vi "Main.vi"() -> ()   [LabVIEW 2014, in "Configurable.lvlib"]
doc: "This template is based off of the Queued Message Handler design pattern and the Queued Message Handler project template that ships with LabVIEW.\n\nThe main difference is that the queue is private to this module and communication between modules is performed via Broadcast and Request events.\n\nRequest events are wrapped in public API methods and are handled in the Event Handling Loop (EHL) of this VI. Any module can register for Broadcast events sent by this module. The EHL generates messages based on user interface actions.\n\nThe Message Handling Loop (MHL) processes messages generated by the EHL, or by other messages. The messages are string values, so new messages can be added easily to the Message Cases case structure in the MHL. Each message cluster can also provide an optional value for Message Data, which is a variant that can be converted to whatever message-specific data is required.\n_____\nBased on Delacor QMH Project Template 4.0.0.47."
uses:
  Configurable.lvlib
  <vilib>/Delacor/Delacor QMH/Libraries/Cloneable Module Admin_class/Delacor_lib_QMH_Cloneable Module Admin.lvclass
  <vilib>/LabVIEW Open Source/Configuration Manager/Manager/ConfigManager.lvclass
  <vilib>/LabVIEW Open Source Project/Unicity/UniqueName/UniqueNameClass/UniqueName.lvclass
  ModuleConfiguration--Cluster.ctl
  Module Data--cluster.ctl
  <vilib>/Delacor/Delacor QMH/Libraries/Cloneable Module Admin_class/Delacor_lib_QMH_Cloneable Module Admin.lvclass/Delacor_lib_QMH_Cloneable Module Admin.ctl
  Stop Argument--cluster.ctl
  <vilib>/Delacor/Delacor QMH/Libraries/Module Admin_class/Delacor_lib_QMH_Module Admin.lvclass/Delacor_lib_QMH_Module Admin.ctl
  GetQualifiedName Argument--cluster.ctl
  GetQualifiedName (Reply Payload)--cluster.ctl
  GetConfiguration Argument--cluster.ctl
  GetConfiguration (Reply Payload)--cluster.ctl
  Modify Configuration Argument--cluster.ctl
  <vilib>/Utility/miscctls.llb/LVPointTypeDef.ctl
  <vilib>/LabVIEW Open Source Project/Unicity/UniqueName/UniqueNameClass/UniqueName.lvclass/UniqueName.ctl
  <vilib>/Delacor/Delacor QMH/Libraries/Cloneable Module Admin_class/Delacor_lib_QMH_Get Module ID.vi
  <vilib>/Delacor/Delacor QMH/Libraries/Module Admin_class/Delacor_lib_QMH_Get External Launch.vi
  <vilib>/Delacor/Delacor QMH/Libraries/Message Queue_class/Delacor_lib_QMH_Enqueue Message (Single).vi
  <vilib>/Utility/error.llb/Error Cluster From Error Code.vi
  <vilib>/ErrorRing/Error Ring.xnode
  <vilib>/Delacor/Delacor QMH/Libraries/Message Queue_class/Delacor_lib_QMH_Message Queue.lvclass
  Clone Registration/Clone Registration.lvlib
panel:
  out "Initial Configuration":T1
  out "Current Configuration":T1
  in  "Self":refnum<class "UniqueName.lvclass">
  in  "CfgManager":refnum<class "ConfigManager.lvclass">
  in  "Simulate MHL Error":bool
  in  "Simulate EHL Error":bool
  out "error out":errorcluster
  in  "Module Admin":refnum<class "Delacor_lib_QMH_Cloneable Module Admin.lvclass">
  out "Status":string
  # "Do not modify these nodes"
  # "This template is for the a Configurable  Delacor Queued Message Handler design pattern.\n\nSee the block diagram for more information on how to use this template.\nOther QMH Modules communicate with this Module via its Public API (wrappers for its Request Events).\n\nThis Module communicates with other Modules via its Broadcast Events.\nAny module that wants to get these messages, just registers for this module's Broadcast events."
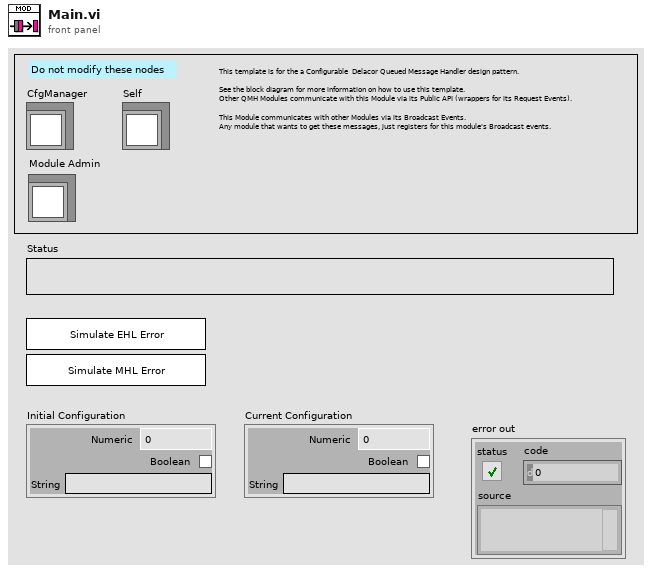
[diagram p1: front panel]
types:
  T1 = typedef "Configurable.lvlib/ModuleConfiguration--Cluster.ctl" = cluster{"Numeric":dbl, "Boolean":bool, "String":string}
  T2 = typedef "Configurable.lvlib/Module Data--cluster.ctl" = cluster{"Status":string, "CfgManager":refnum<class "ConfigManager.lvclass">, "Self":refnum<class "UniqueName.lvclass">}
  T3 = typedef "Configurable.lvlib/Request Events--cluster.ctl" = cluster{"Stop Module":refnum<user-event>, "Show Panel":refnum<user-event>, "Hide Panel":refnum<user-event>, "Show Diagram":refnum<user-event>, "Get Module Execution Status":refnum<user-event>, "GetQualifiedName":refnum<user-event>, "GetConfiguration":refnum<user-event>, "Modify Configuration":refnum<user-event>}
  T4 = enum32{"invalid lock state", "Not Locked", "Locked (No Password)", "Password-protected"}
  T5 = typedef "Configurable.lvlib/Stop Argument--cluster.ctl" = cluster{"Origin":string, "Module ID":i32, "Exit via Stop Module Req?":bool, "Wait for Module to stop?":bool}
  T6 = typedef "Configurable.lvlib/GetQualifiedName Argument--cluster.ctl" = cluster{"Module ID":i32, "Fully Qualified Name":string, "Wait Notifier":refnum<notifier>}
  T7 = typedef "Configurable.lvlib/GetConfiguration Argument--cluster.ctl" = cluster{"Module ID":i32, "Wait Notifier":refnum<notifier>}
  T8 = typedef "Configurable.lvlib/Modify Configuration Argument--cluster.ctl" = cluster{"Module ID":i32, "Configuration":T1}
  T9 = typedef "LVPointTypeDef.ctl" = cluster{"Horizontal":i16, "Vertical":i16}
  T10 = enum32{"Invalid", "Standard", "Closed", "Hidden", "Minimized", "Maximized"}
  T11 = typedef "Configurable.lvlib/GetQualifiedName (Reply Payload)--cluster.ctl" = cluster{"Fully Qualified Name":string, "GetQualifiedName_error":errorcluster}
  T12 = typedef "Configurable.lvlib/GetConfiguration (Reply Payload)--cluster.ctl" = cluster{"Configuration":T1, "GetConfiguration_error":errorcluster}
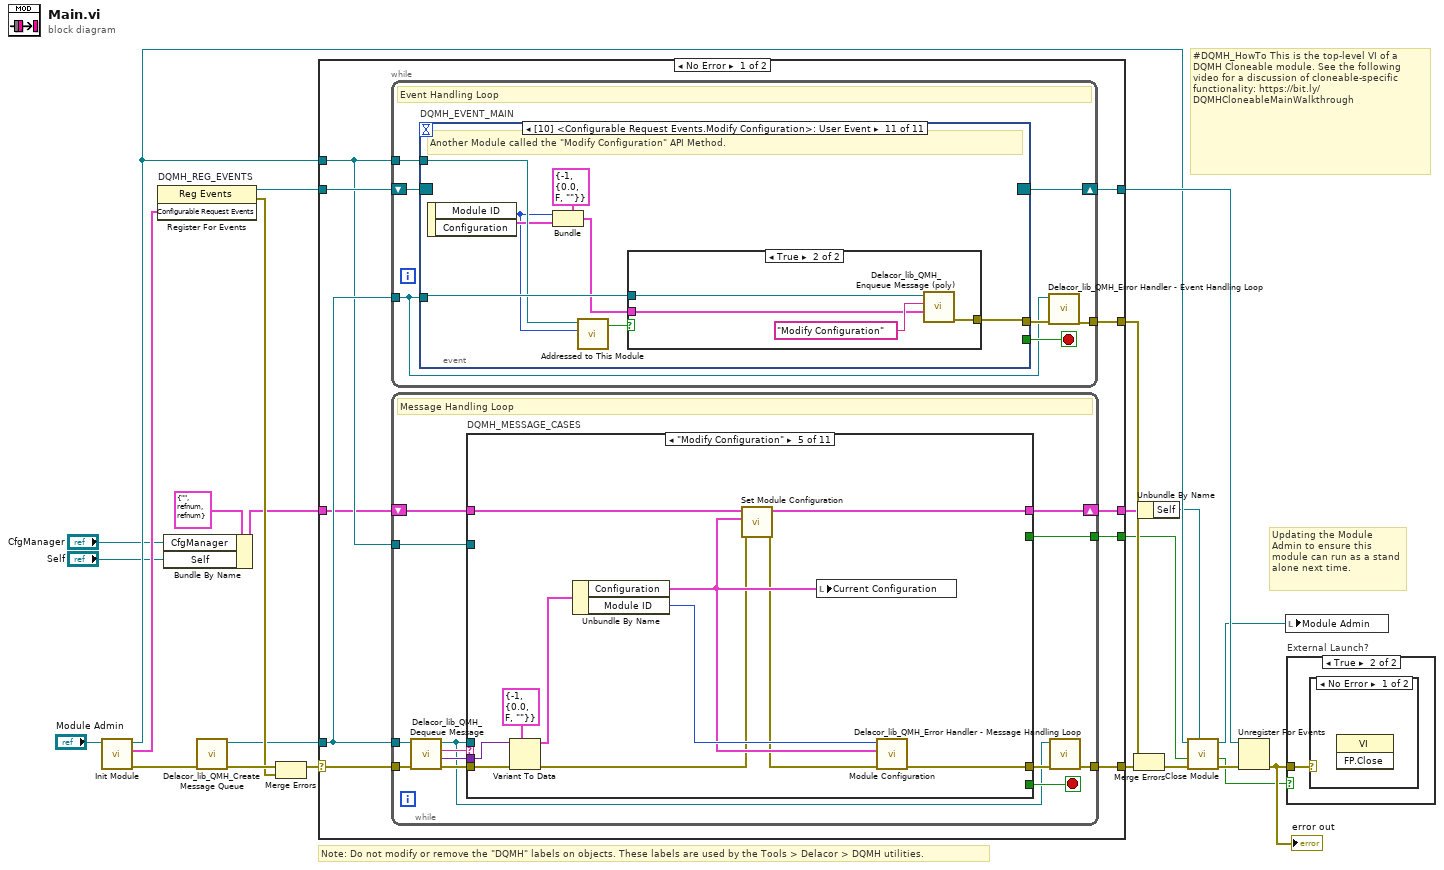
[diagram p0: block diagram]
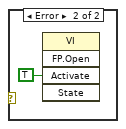
[diagram p3: hidden frame]
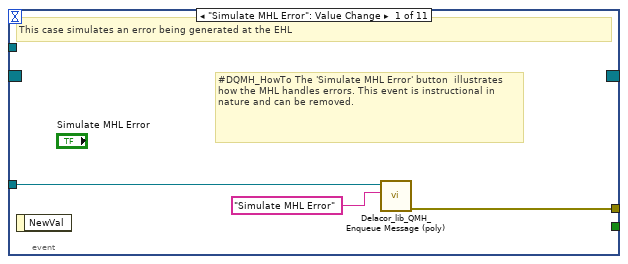
[diagram p4: hidden frame]
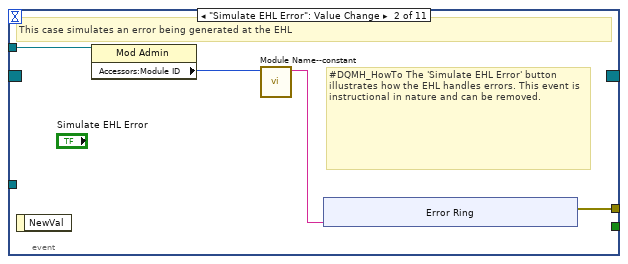
[diagram p5: hidden frame]
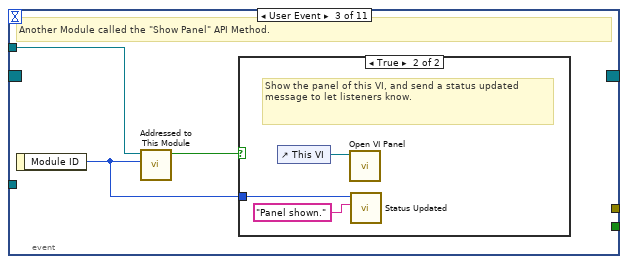
[diagram p6: hidden frame]
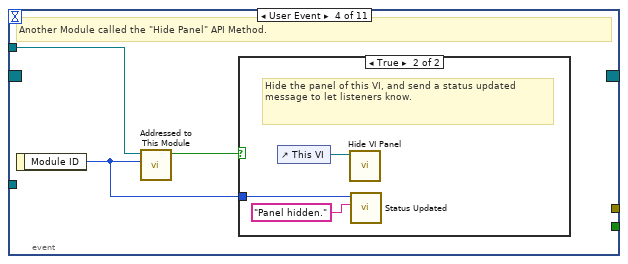
[diagram p8: hidden frame]
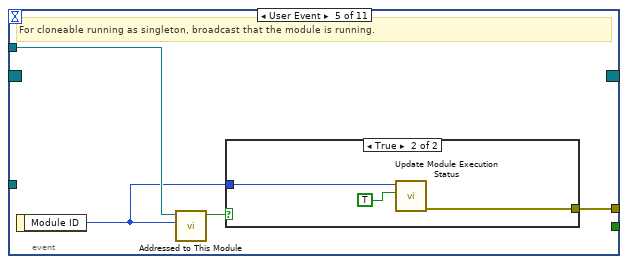
[diagram p10: hidden frame]
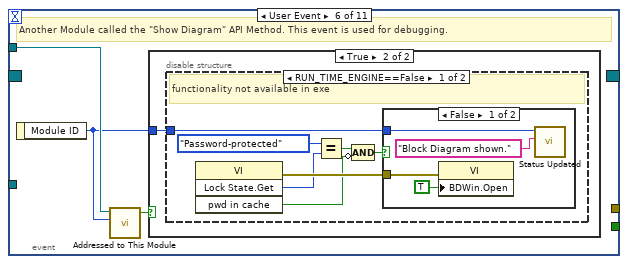
[diagram p12: hidden frame]
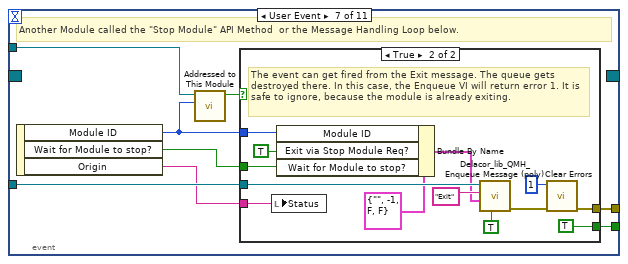
[diagram p16: hidden frame]
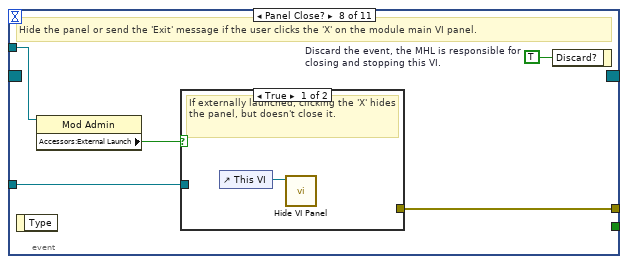
[diagram p18: hidden frame]
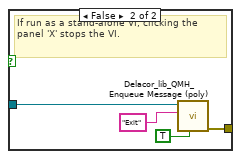
[diagram p19: hidden frame]
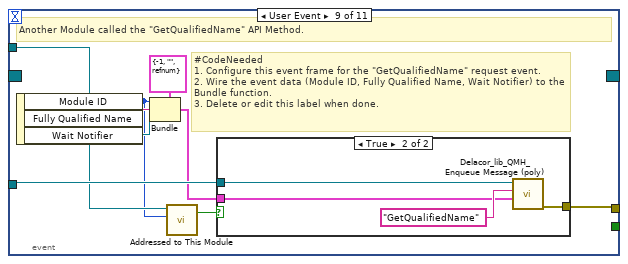
[diagram p20: hidden frame]
diagram:
  # "#DQMH_HowTo This is the top-level VI of a DQMH Cloneable module. See the following video for a discussion of cloneable-specific functionality: https://bit.ly/DQMHCloneableMainWalkthrough"
  # "Note: Do not modify or remove the \"DQMH\" labels on objects. These labels are used by the Tools > Delacor > DQMH utilities."
  # "Updating the Module Admin to ensure this module can run as a stand alone next time."
  n1 = call "Init Module.vi"("Cloneable Module Admin in"="Module Admin") -> ("error out"=w21:errorcluster, "Configurable Request Events"=w13:T3, "Cloneable Module Admin out"=w10:refnum<class "Delacor_lib_QMH_Cloneable Module Admin.lvclass">)  [unwired: 8 in]
  n2 = register-events "DQMH_REG_EVENTS"(w13) -> (reference out=w14:refnum<event-registration>, error out=w16:errorcluster)  [unwired: 2 in]
  n3 = Bundle By Name(cluster=T2 {"Status"="", "CfgManager"=refnum, "Self"=refnum} ("Data Cluster"), "CfgManager"="CfgManager", "Self"="Self") -> (w4:T2)
  n4 = call <vilib>:"Delacor_lib_QMH_Create Message Queue.vi"("error in (no error)"=w21) -> ("error out"=w18:errorcluster, "Message Queue out"=w12:refnum<class "Delacor_lib_QMH_Message Queue.lvclass">)  [unwired: 9 in]
  n5 = Merge Errors(w18, w16) -> (w17:errorcluster)
  n6 = case shown="No Error" w17 {
    selector: w17 -> [w32 w317]
    tunnel: [w34 w317] -> w22
    tunnel: [w31 w316] -> w15
    tunnel: w14 -> [w30 w316]
    tunnel: w12 -> [w29 _]
    tunnel: [w33 _] -> w23
    tunnel: w10 -> [w28 w312]
    tunnel: [w27 _] -> w8
    tunnel: w4 -> [w26 w309]
    tunnel: [w25 w309] -> w2
    frame No Error {
      n7 = while {
        tunnel: w29 -> [w35]
        shift-right: [w38] -> w31
        shift-left: w30 -> [w39]
        tunnel: [w40] -> w33
        tunnel: w28 -> [w36]
        stop <- w37 stop-if-true
        # "Event Handling Loop"
        n8 = event "DQMH_EVENT_MAIN" shown="[10] <Configurable Request Events.Modify Configuration>: User Event" {
          selector: w39 -> [_ _ _ _ _ _ _ _ _ _ _]
          dyn-events: [_ _ _ _ _ _ _ _ _ _ _] -> w38
          timeout: _ -> [_ _ _ _ _ _ _ _ _ _ _]
          tunnel: [_ _ _ _ _ _ w93 _ _ _ _] -> w37
          tunnel: w35 -> [w43 _ _ _ _ _ w96 w112 w129 w141 w153]
          tunnel: [w44 w48 _ _ w71 _ w97 w115 w124 w136 w148] -> w41
          tunnel: w36 -> [_ w47 w57 w63 w69 w76 w95 w113 w127 w139 w151]
          event "Simulate MHL Error": Value Change {
            # "#DQMH_HowTo The 'Simulate MHL Error' button  illustrates how the MHL handles errors. This event is instructional in nature and can be removed."
            # "This case simulates an error being generated at the EHL"
            n9 = event-data() -> ()  [unwired: 1 in, 1 out]
            n10 = call-poly <vilib>:"Delacor_lib_QMH_Enqueue Message (poly).vi"("Message"="Simulate MHL Error", "Message Queue in"=w43) -> ("error out"=w44:errorcluster)  [unwired: 8 in, 1 out]
          }
          event "Simulate EHL Error": Value Change {
            # "#DQMH_HowTo The 'Simulate EHL Error' button  illustrates how the EHL handles errors. This event is instructional in nature and can be removed."
            # "This case simulates an error being generated at the EHL"
            n11 = event-data() -> ()  [unwired: 1 in, 1 out]
            n12 = property class="Mod Admin"(reference=w47) -> ("Accessors:Module ID"=w46:i32)  [unwired: 1 in, 2 out]
            n13 = call "Module Name--constant.vi"("Module ID"=w46) -> ("Module Name"=w45:string)  [unwired: 10 in]
            n14 = xnode "Error Ring"("parameter 0"=w45) -> ("error out"=w48:errorcluster)
          }
          event User Event {
            # "Another Module called the \"Show Panel\" API Method."
            n15 = event-data() -> ("Module ID"=w56:i32)  [unwired: 1 in]
            n16 = call "Addressed to This Module.vi"("Module ID from Argument"=w56, "Module Admin"=w57) -> ("Addressed to this instance?"=w58:bool)  [unwired: 8 in, 1 out]
            n17 = case shown="True" w58 {
              tunnel: w56 -> [_ w59]
              frame False {
              }
              frame True {
                # "Show the panel of this VI, and send a status updated message to let listeners know."
                n18 = control-ref of="This VI"() -> (w61:refnum<vi>)
                n19 = call "Open VI Panel.vi"("VI"=w61) -> ()  [unwired: 10 in, 1 out]
                n20 = call "Status Updated.vi"("Status"="Panel shown." ("format string"), "Module ID"=w59) -> ()  [unwired: 9 in, 1 out]
              }
            }
          }
          event User Event {
            # "Another Module called the \"Hide Panel\" API Method."
            n21 = event-data() -> ("Module ID"=w62:i32)  [unwired: 1 in]
            n22 = call "Addressed to This Module.vi"("Module ID from Argument"=w62, "Module Admin"=w63) -> ("Addressed to this instance?"=w64:bool)  [unwired: 8 in, 1 out]
            n23 = case shown="True" w64 {
              tunnel: w62 -> [_ w65]
              frame False {
              }
              frame True {
                # "Hide the panel of this VI, and send a status updated message to let listeners know."
                n24 = control-ref of="This VI"() -> (w67:refnum<vi>)
                n25 = call "Hide VI Panel.vi"("VI"=w67) -> ()  [unwired: 10 in, 1 out]
                n26 = call "Status Updated.vi"("Status"="Panel hidden." ("format string"), "Module ID"=w65) -> ()  [unwired: 9 in, 1 out]
              }
            }
          }
          event User Event {
            # "For cloneable running as singleton, broadcast that the module is running."
            n27 = event-data() -> ("Module ID"=w68:i32)  [unwired: 1 in]
            n28 = call "Addressed to This Module.vi"("Module ID from Argument"=w68, "Module Admin"=w69) -> ("Addressed to this instance?"=w70:bool)  [unwired: 8 in, 1 out]
            n29 = case shown="True" w70 {
              tunnel: [_ w74] -> w71
              tunnel: w68 -> [_ w73]
              frame False {
              }
              frame True {
                n30 = call "Update Module Execution Status.vi"("Running?"=TRUE, "Module ID"=w73) -> ("error out"=w74:errorcluster)  [unwired: 9 in]
              }
            }
          }
          event User Event {
            # "Another Module called the \"Show Diagram\" API Method. This event is used for debugging."
            n31 = event-data() -> ("Module ID"=w75:i32)  [unwired: 1 in]
            n32 = call "Addressed to This Module.vi"("Module ID from Argument"=w75, "Module Admin"=w76) -> ("Addressed to this instance?"=w77:bool)  [unwired: 8 in, 1 out]
            n33 = case shown="True" w77 {
              tunnel: w75 -> [_ w78]
              frame False {
              }
              frame True {
                n34 = disable-structure shown="RUN_TIME_ENGINE==False" {
                  disable-tunnel: w78 -> [w79 _]
                  frame condition #0 (active) {
                    # "functionality not available in exe"
                    n35 = invoke class="VI" method="Lock State.Get"() -> (error out=w85:errorcluster, "Get Lock State"=w84:T4, "pwd in cache"=w81:bool)  [unwired: 4 in, 1 out]
                    n36 = Equal?(x=T4."Password-protected", y=w84) -> (x = y?=w82:bool)
                    n37 = Compound Arithmetic op=AND(w82, invert w81) -> (w80:bool)
                    n38 = case shown="False" w80 {
                      tunnel: w85 -> [w89 _]
                      tunnel: w79 -> [w86 _]
                      frame False {
                        n39 = property class="VI"(error in=w89, "BDWin.Open"=TRUE ("Block Diagram Window:Open")) -> ()  [unwired: 1 in, 2 out]
                        n40 = call "Status Updated.vi"("Status"="Block Diagram shown." ("format string"), "Module ID"=w86) -> ()  [unwired: 9 in, 1 out]
                      }
                      frame True {
                        # "Password-protected VI, and the password is not in the cache. Do not show the diagram."
                      }
                    }
                  }
                  frame condition #1 {
                  }
                }
              }
            }
          }
          event User Event {
            # "Another Module called the \"Stop Module\" API Method  or the Message Handling Loop below."
            n41 = event-data() -> ("Module ID"=w91:i32, "Wait for Module to stop?"=w92:bool, "Origin"=w90:string)  [unwired: 1 in]
            n42 = call "Addressed to This Module.vi"("Module ID from Argument"=w91, "Module Admin"=w95) -> ("Addressed to this instance?"=w94:bool)  [unwired: 8 in, 1 out]
            n43 = case shown="True" w94 {
              tunnel: [_ w109] -> w97
              tunnel: w96 -> [_ w105]
              tunnel: [_ TRUE] -> w93
              tunnel: w92 -> [_ w100]
              tunnel: w91 -> [_ w102]
              tunnel: w90 -> [_ w98]
              frame False {
              }
              frame True {
                # "The event can get fired from the Exit message. The queue gets destroyed there. In this case, the Enqueue VI will return error 1. It is safe to ignore, because the module is already exiting."
                n44 = local write "Status"(w98) -> ()
                n45 = Bundle By Name(cluster=T5 {"Origin"="", "Module ID"=-1, "Exit via Stop Module Req?"=FALSE, "Wait for Module to stop?"=FALSE} ("Stop Argument"), "Module ID"=w102, "Exit via Stop Module Req?"=TRUE, "Wait for Module to stop?"=w100) -> (w99:T5)
                n46 = call-poly <vilib>:"Delacor_lib_QMH_Enqueue Message (poly).vi"("Priority Message? (F)"=TRUE, "Message Data"=w99, "Message"="Exit", "Message Queue in"=w105) -> ("error out"=w110:errorcluster)  [unwired: 6 in, 1 out]
                n47 = call <vilib>:"Clear Errors.vi"("error in (no error)"=w110, "specific error code to clear (0: all)"=1) -> ("error out"=w109:errorcluster)  [unwired: 4 in, 1 out]
              }
            }
          }
          event Panel Close? {
            w114 = TRUE  # Discard the event, the MHL is responsible for closing and stopping this VI.
            # "Hide the panel or send the 'Exit' message if the user clicks the 'X' on the module main VI panel."
            n48 = event-data() -> ()  [unwired: 1 in, 1 out]
            n49 = property class="Mod Admin"(reference=w113) -> ("Accessors:External Launch"=w111:bool)  [unwired: 1 in, 2 out]
            n50 = case shown="True" w111 {
              tunnel: w112 -> [_ w119]
              tunnel: [_ w120] -> w115
              frame True {
                # "If externally launched, clicking the 'X' hides the panel, but doesn't close it."
                n51 = control-ref of="This VI"() -> (w116:refnum<vi>)
                n52 = call "Hide VI Panel.vi"("VI"=w116) -> ()  [unwired: 10 in, 1 out]
              }
              frame False {
                # "If run as a stand-alone VI, clicking the panel 'X' stops the VI."
                n53 = call-poly <vilib>:"Delacor_lib_QMH_Enqueue Message (poly).vi"("Priority Message? (F)"=TRUE, "Message"="Exit", "Message Queue in"=w119) -> ("error out"=w120:errorcluster)  [unwired: 7 in, 1 out]
              }
            }
            n54 = event-data("Discard?"=w114) -> ()  [unwired: 1 in, 1 out]
          }
          event User Event {
            # "#CodeNeeded\n1. Configure this event frame for the \"GetQualifiedName\" request event.\n2. Wire the event data (Module ID, Fully Qualified Name, Wait Notifier) to the Bundle function.\n3. Delete or edit this label when done."
            # "Another Module called the \"GetQualifiedName\" API Method."
            n55 = event-data() -> ("Module ID"=w121:i32, "Fully Qualified Name"=w123:string, "Wait Notifier"=w122:refnum<notifier>)  [unwired: 1 in]
            n56 = Bundle(cluster=T6 {"Module ID"=-1, "Fully Qualified Name"="", "Wait Notifier"=refnum} ("GetQualifiedName Argument"), "Module ID"=w121, "Fully Qualified Name"=w123, "Wait Notifier"=w122) -> (w125:T6)
            n57 = call "Addressed to This Module.vi"("Module ID from Argument"=w121, "Module Admin"=w127) -> ("Addressed to this instance?"=w128:bool)  [unwired: 8 in, 1 out]
            n58 = case shown="True" w128 {
              tunnel: w129 -> [_ w133]
              tunnel: w125 -> [_ w131]
              tunnel: [_ w130] -> w124
              frame False {
              }
              frame True {
                n59 = call-poly <vilib>:"Delacor_lib_QMH_Enqueue Message (poly).vi"("Message Data"=w131, "Message"="GetQualifiedName", "Message Queue in"=w133) -> ("error out"=w130:errorcluster)  [unwired: 7 in, 1 out]
              }
            }
          }
          event User Event {
            # "Another Module called the \"GetConfiguration\" API Method."
            n60 = event-data() -> ("Module ID"=w134:i32, "Wait Notifier"=w135:refnum<notifier>)  [unwired: 1 in]
            n61 = Bundle(cluster=T7 {"Module ID"=-1, "Wait Notifier"=refnum} ("GetConfiguration Argument"), "Module ID"=w134, "Wait Notifier"=w135) -> (w137:T7)
            n62 = call "Addressed to This Module.vi"("Module ID from Argument"=w134, "Module Admin"=w139) -> ("Addressed to this instance?"=w140:bool)  [unwired: 8 in, 1 out]
            n63 = case shown="True" w140 {
              tunnel: w141 -> [_ w145]
              tunnel: w137 -> [_ w143]
              tunnel: [_ w142] -> w136
              frame False {
              }
              frame True {
                n64 = call-poly <vilib>:"Delacor_lib_QMH_Enqueue Message (poly).vi"("Message Data"=w143, "Message"="GetConfiguration", "Message Queue in"=w145) -> ("error out"=w142:errorcluster)  [unwired: 7 in, 1 out]
              }
            }
          }
          event User Event {
            # "Another Module called the \"Modify Configuration\" API Method."
            n65 = event-data() -> ("Module ID"=w146:i32, "Configuration"=w147:T1)  [unwired: 1 in]
            n66 = Bundle(cluster=T8 {"Module ID"=-1, "Configuration"={"Numeric"=0.0, "Boolean"=FALSE, "String"=""}} ("Modify Configuration Argument"), "Module ID"=w146, "Configuration"=w147) -> (w149:T8)
            n67 = call "Addressed to This Module.vi"("Module ID from Argument"=w146, "Module Admin"=w151) -> ("Addressed to this instance?"=w152:bool)  [unwired: 8 in, 1 out]
            n68 = case shown="True" w152 {
              tunnel: w153 -> [_ w157]
              tunnel: w149 -> [_ w155]
              tunnel: [_ w154] -> w148
              frame False {
              }
              frame True {
                n69 = call-poly <vilib>:"Delacor_lib_QMH_Enqueue Message (poly).vi"("Message Data"=w155, "Message"="Modify Configuration", "Message Queue in"=w157) -> ("error out"=w154:errorcluster)  [unwired: 7 in, 1 out]
              }
            }
          }
        }
        n70 = call-dynamic "Delacor_lib_QMH_Error Handler - Event Handling Loop.vi"("error in (no error)"=w41, "Message Queue in"=w35) -> ("dup error in"=w40:errorcluster)  [unwired: 8 in, 1 out]
      }
      n71 = while {
        tunnel: w29 -> [w161]
        shift-right: [w165] -> w25
        shift-left: w26 -> [w166]
        tunnel: w32 -> [w169]
        tunnel: [w167] -> w34
        tunnel: w28 -> [w159]
        tunnel: [w158] -> w27
        stop <- w164 stop-if-true
        # "Message Handling Loop"
        n72 = call-dynamic "Delacor_lib_QMH_Dequeue Message.vi"("error in (no error)"=w169, "Message Queue in"=w161) -> ("error out"=w168:errorcluster, "Message Data"=w162:variant, "Message"=w163:string, "Message Queue out"=w160:refnum<class "Delacor_lib_QMH_Message Queue.lvclass">)  [unwired: 6 in]
        n73 = case "DQMH_MESSAGE_CASES" shown="\"Modify Configuration\"" w163 {
          selector: w163 -> [_ _ _ _ _ _ _ _ _ _ w296]
          tunnel: w160 -> [_ _ _ _ _ _ _ w246 _ w286 _]
          tunnel: w168 -> [w197 w201 w217 w229 w240 w243 w245 w256 w269 w292 w298]
          tunnel: [w179 w201 w206 w221 w234 w242 w245 w252 w268 w289 w299] -> w170
          tunnel: w166 -> [w173 w200 w211 w220 w236 w241 w244 w251 w266 w285 w297]
          tunnel: [w189 w200 w211 w219 w235 w241 w244 w251 w266 w285 w297] -> w165
          tunnel: [_ _ _ _ _ _ _ _ _ w284 _] -> w164
          tunnel: w162 -> [_ _ w216 w228 w239 _ _ w250 _ w282 _]
          tunnel: w159 -> [w185 _ _ _ _ _ _ w249 w264 w278 w294]
          tunnel: [_ _ _ _ _ _ _ _ _ w280 _] -> w158
          frame "Initialize" {
            w183 = "Initial Message" ("Initial Message")
            # "THIS OVERRIDES THE\nCONFIG FOR DEMO PURPOSES.\nREMOVE IT."
            # "Initialize - Any operation that needs to be done before the module can receive messages. Synchronize Caller Events.vi will inform Start Module.vi that the module has launched and is ready to receive messages. Module Did Init.vi will broadcast that the module initialized."
            n74 = call "Synchronize Caller Events.vi"("error in (no error)"=w197, "Module Admin"=w185) -> ("error out"=w196:errorcluster, "Module Admin out"=w174:refnum<class "Delacor_lib_QMH_Cloneable Module Admin.lvclass">)  [unwired: 8 in]
            n75 = Unbundle By Name(w173) -> ("Self"=w172:refnum<class "UniqueName.lvclass">)
            n76 = call <vilib>:"Read UUID.vi"("UniqueName in"=w172) -> ("UUID"=w171:string)  [unwired: 9 in, 1 out]
            n77 = property class="Mod Admin"(reference=w174) -> ("Accessors:Module ID"=w178:i32, "Accessors:External Launch"=w186:bool)  [unwired: 1 in, 2 out]
            n78 = Random Number (0-1)() -> (number: 0 to 1=w182:dbl)
            n79 = call "Get Module Configuration.vi"("Data Cluster"=w173) -> ("Configuration"=w181:T1, "Data Cluster dup"=w177:T2)  [unwired: 8 in, 1 out]
            n80 = Bundle By Name(cluster=w181, "Numeric"=w182, "String"=w171) -> (w175:T1)
            "Initial Configuration" <- w175
            n81 = call "Module Name--constant.vi"("Module ID"=w178) -> ("Module Name"=w193:string)  [unwired: 10 in]
            n82 = local write "Current Configuration"(w175) -> ()
            n83 = call "Set Module Configuration.vi"("Configuration"=w175, "Data Cluster"=w177) -> ("Data Cluster dup"=w176:T2)  [unwired: 8 in, 1 out]
            n84 = call "Module Name--constant.vi"("Module ID"=w178) -> ("Module Name"=w187:string)  [unwired: 10 in]
            n85 = property class="VI"("Front Panel.Title"=w193) -> (reference out=w195:refnum<vi>, error out=w199:errorcluster)  [unwired: 2 in]
            n86 = Select(t=T10."Hidden" ("State"), s=w186, f=T10."Standard" ("State")) -> (s? t:f=w190:T10)
            n87 = call "Module Did Init.vi"("error in (no error)"=w196, "Initialized?"=TRUE, "Origin"=w187, "Module ID"=w178) -> ("error out"=w180:errorcluster)  [unwired: 7 in]
            n88 = invoke class="VI" method="FP.Open"(reference=w195, error in=w199, "State"=w190) -> (reference out=w194:refnum<vi>, error out=w198:errorcluster)  [unwired: 2 in, 3 out]
            n89 = Bundle By Name(cluster=w176, "Status"=w183) -> (w189:T2)
            n90 = invoke class="VI" method="FP.Center"(reference=w194, error in=w198) -> ()  [unwired: 1 in, 3 out]
            n91 = property on="Pane" class="Pane"("Origin"=T9 {"Horizontal"=0, "Vertical"=0}) -> ()  [unwired: 2 in, 2 out]
            n92 = call "Module Configuration.vi"("error in (no error)"=w180, "Configuration"=w175, "Module ID"=w178) -> ("error out"=w179:errorcluster)  [unwired: 8 in]
            "Status" <- w183
          }
          frame "--- Module Specific ---" {
            # "Separator -- The following cases handle messages specific to this Module."
          }
          frame "GetQualifiedName" {
            # "Requests the module's Fully Qualified Name"
            n93 = Unbundle By Name(w211) -> ("Self"=w210:refnum<class "UniqueName.lvclass">)
            n94 = Variant To Data(error in=w217, type=T6 {"Module ID"=-1, "Fully Qualified Name"="", "Wait Notifier"=refnum} ("GetQualifiedName Argument"), Variant=w216) -> (data=w214:T6, error out=w205:errorcluster)
            n95 = call <vilib>:"Read Fully Qualified Name.vi"("UniqueName in"=w210) -> ("Fully Qualified Name"=w204:string)  [unwired: 9 in, 1 out]
            n96 = Unbundle By Name(w214) -> ("Wait Notifier"=w212:refnum<notifier>, "Module ID"=w208:i32)
            n97 = Bundle By Name(cluster=T11 {"Fully Qualified Name"="", "GetQualifiedName_error"={"status"=FALSE, "code"=0, "source"=""}} ("GetQualifiedName (Reply Payload)"), "Fully Qualified Name"=w204) -> (w213:T11)
            n98 = Format Into String(format string="FQN: %s", w204) -> (resulting string=w203:string)  [unwired: 2 in, 1 out]
            n99 = Send Notification(notification=w213, notifier=w212, error in (no error)=w205) -> (error out=w207:errorcluster)  [unwired: 1 out]
            n100 = call "Status Updated.vi"("error in (no error)"=w207, "Status"=w203, "Module ID"=w208) -> ("error out"=w206:errorcluster)  [unwired: 8 in]
          }
          frame "GetConfiguration" {
            n101 = Variant To Data(error in=w229, type=T7 {"Module ID"=-1, "Wait Notifier"=refnum} ("GetConfiguration Argument"), Variant=w228) -> (data=w226:T7, error out=w222:errorcluster)
            n102 = call "Get Module Configuration.vi"("error in (no error)"=w222, "Data Cluster"=w220) -> ("error out"=w221:errorcluster, "Configuration"=w218:T1, "Data Cluster dup"=w219:T2)  [unwired: 7 in]
            "Current Configuration" <- w218
            n103 = Unbundle By Name(w226) -> ("Wait Notifier"=w225:refnum<notifier>)
            n104 = Bundle By Name(cluster=T12 {"Configuration"={"Numeric"=0.0, "Boolean"=FALSE, "String"=""}, "GetConfiguration_error"={"status"=FALSE, "code"=0, "source"=""}} ("GetConfiguration (Reply Payload)"), "Configuration"=w218, "GetConfiguration_error"=w221) -> (w224:T12)
            n105 = Send Notification(notification=w224, notifier=w225) -> ()  [unwired: 1 in, 2 out]
          }
          frame "Modify Configuration" {
            n106 = Variant To Data(error in=w240, type=T8 {"Module ID"=-1, "Configuration"={"Numeric"=0.0, "Boolean"=FALSE, "String"=""}} ("Modify Configuration Argument"), Variant=w239) -> (data=w237:T8, error out=w231:errorcluster)
            n107 = Unbundle By Name(w237) -> ("Configuration"=w232:T1, "Module ID"=w233:i32)
            n108 = call "Set Module Configuration.vi"("error in (no error)"=w231, "Configuration"=w232, "Data Cluster"=w236) -> ("error out"=w230:errorcluster, "Data Cluster dup"=w235:T2)  [unwired: 7 in]
            n109 = local write "Current Configuration"(w232) -> ()
            n110 = call "Module Configuration.vi"("error in (no error)"=w230, "Configuration"=w232, "Module ID"=w233) -> ("error out"=w234:errorcluster)  [unwired: 8 in]
          }
          frame "---Copy This Frame---" {
            # "Duplicate this frame when creating new messages.  Change this comment in the duplicated frame to describe this message."
            n111 = Merge Errors(w243) -> (w242:errorcluster)
          }
          frame "--- Exit and Error Handling---" {
            # "Separator - the following cases handle errors and exit messages."
          }
          frame "Error" {
            # "#CodeRecommended - If you ever change the name of this \"Error\" message, you'll need to update the name in the Check Loop Error.vi as well."
            # "#CodeRecommended - If the module is running in standalone mode (External Launch = FALSE), this code will pop up an error dialog and call the 'Exit' message if an error occurs. Add more fine-grained error handling here."
            # "Error - Check the error message data and respond accordingly. This message is sent by the \"Error Handler\" VIs at the end of each loop in this application."
            n112 = property class="Mod Admin"(reference=w249) -> ("Accessors:External Launch"=w247:bool, "Accessors:Module ID"=w248:i32)  [unwired: 1 in, 2 out]
            n113 = Variant To Data(error in=w256, type=errorcluster {"status"=FALSE, "code"=0, "source"=""} ("error constant"), Variant=w250) -> (data=w257:errorcluster, error out=w254:errorcluster)
            n114 = call "Error Reported.vi"("Error"=w257, "Module ID"=w248) -> ()  [unwired: 9 in, 1 out]
            n115 = case shown="False" w247 {
              tunnel: [w262 _] -> w253
              tunnel: w246 -> [w260 _]
              tunnel: w257 -> [w261 _]
              frame False {
                # "If the module is running standalone, then pop up an error dialog and call the \"Exit\" message."
                n116 = call <vilib>:"Simple Error Handler.vi"("error in (no error)"=w261) -> ()  [unwired: 4 in, 5 out]
                n117 = call-poly <vilib>:"Delacor_lib_QMH_Enqueue Message (poly).vi"("Priority Message? (F)"=TRUE, "Message"="Exit", "Message Queue in"=w260) -> ("error out"=w262:errorcluster)  [unwired: 7 in, 1 out]
              }
              frame True {
                # "If the module was launched externally, calling the Error Reported broadcast VI is the only action performed by the \"Error\" message. The module's caller can then process the error appropriately."
              }
            }
            n118 = Merge Errors(w254, w253) -> (w252:errorcluster)
            n119 = local write "error out"(w252) -> ()
          }
          frame "Simulate MHL Error" {
            # "#DQMH_HowTo The 'Simulate MHL Error' button  illustrates how the MHL handles errors. This event is instructional in nature and can be removed."
            # "Simulate an error occurring at the MHL"
            n120 = property class="Mod Admin"(reference=w264) -> ("Accessors:Module ID"=w265:i32)  [unwired: 1 in, 2 out]
            n121 = call "Module Name--constant.vi"("Module ID"=w265) -> ("Module Name"=w263:string)  [unwired: 10 in]
            n122 = xnode "Error Ring"("parameter 0"=w263) -> ("error out"=w267:errorcluster)
            n123 = Merge Errors(w269, w267) -> (w268:errorcluster)
          }
          frame "Exit" {
            w283 = 91  # 91: not all Exit messages will have an argument
            w284 = TRUE  # Stop the VI
            # "Release the message queue reference"
            # "#CodeNeeded - Add any required cleanup code here."
            # "Exit - Exit the application."
            n124 = Variant To Data(error in=w292, type=T5 {"Origin"="", "Module ID"=-1, "Exit via Stop Module Req?"=FALSE, "Wait for Module to stop?"=FALSE} ("Stop Argument"), Variant=w282) -> (data=w279:T5, error out=w287:errorcluster)
            n125 = call <vilib>:"Clear Errors.vi"("error in (no error)"=w287, "specific error code to clear (0: all)"=w283) -> ("error out"=w291:errorcluster)  [unwired: 4 in, 1 out]
            n126 = control-ref of="This VI"() -> (w277:refnum<vi>)
            n127 = call-dynamic "Delacor_lib_QMH_Release Message Queue.vi"("error in (no error)"=w291, "Message Queue"=w286) -> ("error out"=w290:errorcluster)  [unwired: 9 in]
            n128 = call "Handle Exit.vi"("Stop Argument"=w279, "Module Admin in"=w278, "VI reference"=w277) -> ("error out"=w288:errorcluster, "Wait for Stop?"=w280:bool)  [unwired: 7 in]
            n129 = Merge Errors(w290, w288) -> (w289:errorcluster)
          }
          frame Default {
            # "'Default' case only runs if there is a message that isn't defined in any of the other cases.  Output a programming error."
            n130 = property class="Mod Admin"(reference=w294) -> ("Accessors:Module ID"=w293:i32)  [unwired: 1 in, 2 out]
            n131 = call "Module Name--constant.vi"("Module ID"=w293) -> ("Module Name"=w295:string)  [unwired: 10 in]
            n132 = xnode "Error Ring"("parameter 0"=w296, "parameter 1"=w295) -> ("error out"=w300:errorcluster)
            n133 = Merge Errors(w298, w300) -> (w299:errorcluster)
          }
        }
        n134 = call-dynamic "Delacor_lib_QMH_Error Handler - Message Handling Loop.vi"("error in (no error)"=w170, "Message Queue in"=w160) -> ("dup error in"=w167:errorcluster)  [unwired: 8 in, 1 out]
      }
    }
    frame Error {
      n135 = call "Synchronize Caller Events.vi"("Module Admin"=w312) -> ("Module Admin out"=w311:refnum<class "Delacor_lib_QMH_Cloneable Module Admin.lvclass">)  [unwired: 9 in, 1 out]
      n136 = property class="Mod Admin"(reference=w311) -> ("Accessors:Module ID"=w310:i32)  [unwired: 1 in, 2 out]
      n137 = call "Module Name--constant.vi"("Module ID"=w310) -> ("Module Name"=w315:string)  [unwired: 10 in]
      n138 = call "Remove.vi"("Module ID"=w310) -> ()  [unwired: 9 in, 2 out]
      n139 = Format Into String(format string="An error occurred during initialization. %s is no longer running.", w315) -> (resulting string=w313:string)  [unwired: 2 in, 1 out]
      n140 = call "Error Reported.vi"("Additional Information"=w313, "Error"=w317, "Module ID"=w310) -> ()  [unwired: 8 in, 1 out]
    }
  }
  n141 = Merge Errors(w23, w22) -> (w24:errorcluster)
  n142 = Unbundle By Name(w2) -> ("Self"=w1:refnum<class "UniqueName.lvclass">)
  n143 = call "Close Module.vi"("Self"=w1, "error in (no error)"=w24, "Wait for stop?"=w8, "Module Admin in"=w10) -> ("error out"=w20:errorcluster, "External Launch"=w7:bool, "Module Admin out"=w9:refnum<class "Delacor_lib_QMH_Cloneable Module Admin.lvclass">)  [unwired: 5 in]
  n144 = Unregister For Events(event registration refnum=w15, error in=w20) -> (error out=w19:errorcluster)
  "error out" <- w19
  n145 = local write "Module Admin"(w9) -> ()
  n146 = case "External Launch?" shown="True" w7 {
    tunnel: w19 -> [_ w318]
    frame False {
    }
    frame True {
      n147 = case shown="No Error" w318 {
        frame No Error {
          n148 = invoke class="VI" method="FP.Close"() -> ()  [unwired: 3 in, 3 out]
        }
        frame Error {
          n149 = invoke class="VI" method="FP.Open"("Activate"=TRUE ("Activate?")) -> ()  [unwired: 4 in, 5 out]
        }
      }
    }
  }
